vi "LEBITplc.PressureSafety.vi"(0 "i ref in":refnum<vi>, 1 "Nickname in":string, 2 "i attribute in":T1, 3 "value":dbl, 4 "index in":i32, 5 "error in":errorcluster) -> (14 "i ref out":refnum<vi>, 15 "Nickname out":string, 16 "i attribute out":T1, 17 "value out":dbl, 18 "index out":i32, 19 "error out":errorcluster)   [LabVIEW 2014, in "LEBITplc.lvlib"]
uses:
  LEBITplc.lvlib
  LEBITplc.i attribute.ctl
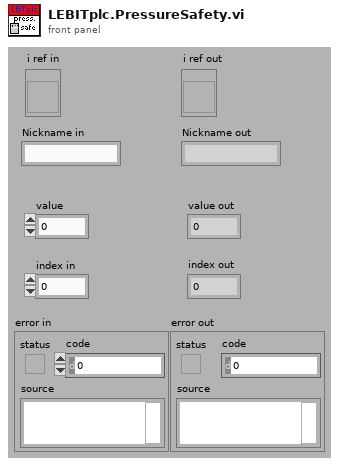
[diagram p1: front panel]
types:
  T1 = typedef "LEBITplc.lvlib/LEBITplc.i attribute.ctl" = cluster{"LLFLocation":string, "SetFileLocation":string, "nickNames":string[], "setValuePLCServiceID":i32[], "GUIServiceID":i32[], "monValuePLC":string[], "SetValueServiceID":i32[], "MonValueServiceID":i32[], "SetValue":dbl[][], "SetValueMin":dbl[], "SetValueMax":dbl[], "SetValueInfoServiceID":i32[], "GUINames":string[], "ListOfBases":string[], "Scale":dbl[], "Offset":dbl[], "setValuePLC":string[], "BaseName":string[], "ScaleServiceID":i32[], "OffsetServiceID":i32[], "AllPLCValues":string[], "CondSpecialArray":string[][], "CondSpecialIndex":i32[], "CondSpecialMonValue":dbl[], "RecentlyChanged":i32[], "SetFileLocationID":i32, "Dependent-Monitors":string[][], "LastLoadedFiles":string[], "IonGuideCalibLocation":string, "Monitor Dependent":string[], "Special":string[], "PLC?":bool[], "Start Date":string, "ListOfBasesServiceID":i32, "SETRA VISA resource":refnum<visa-resource-name>}
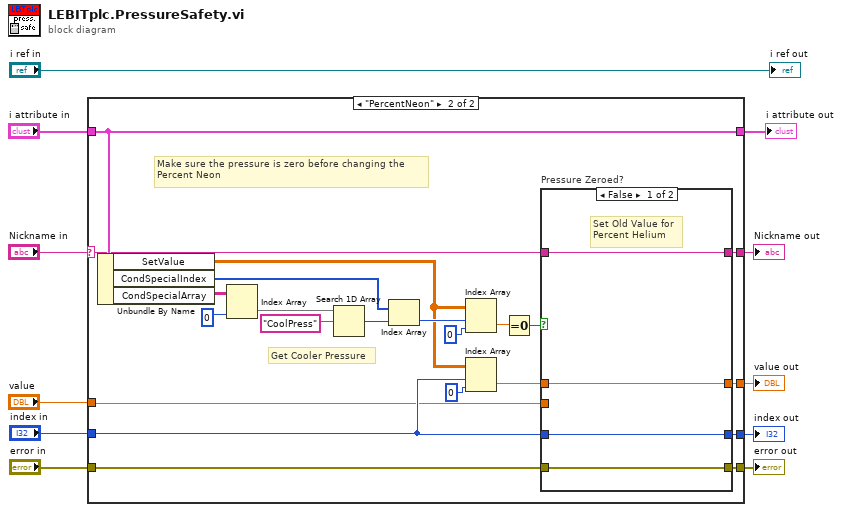
[diagram p0: block diagram]
diagram:
  n1 = case shown="\"PercentNeon\"" "Nickname in" {
    selector: "Nickname in" -> [w14 w34]
    tunnel: "i attribute in" -> [w16 w38]
    tunnel: [w16 w38] -> w9
    tunnel: "value" -> [w13 w20]
    tunnel: [w13 w35] -> w3
    tunnel: [w14 w33] -> w4
    tunnel: "index in" -> [w12 w24]
    tunnel: [w12 w27] -> w2
    tunnel: [w15 w18] -> w5
    tunnel: "error in" -> [w15 w17]
    frame Default {
    }
    frame "PercentNeon" {
      # "Get Cooler Pressure"
      # "Make sure the pressure is zero before changing the \nPercent Neon"
      n2 = Unbundle By Name(w38) -> ("SetValue"=w23:dbl[][], "CondSpecialIndex"=w28:i32[], "CondSpecialArray"=w31:string[][])
      n3 = Index Array(array=w31, index (col)=0 ("index (row)")) -> (element=w32:string[])  [unwired: 1 in]
      n4 = Search 1D Array(1D array=w32, element="CoolPress") -> (index of element=w30:i32)  [unwired: 1 in]
      n5 = Index Array(array=w28, index=w30) -> (element=w29:i32)
      n6 = Index Array(array=w23, index (row)=w29, index (col)=0 ("disabled index (col)")) -> (element=w22:dbl)
      n7 = Index Array(array=w23, index (row)=w24, index (col)=0 ("disabled index (col)")) -> (element=w19:dbl)
      n8 = Equal To 0?(x=w22) -> (x = 0?=w21:bool)
      n9 = case "Pressure Zeroed?" shown="False" w21 {
        tunnel: w20 -> [_ w44]
        tunnel: [w41 w44] -> w35
        tunnel: w34 -> [w40 w45]
        tunnel: [w40 w45] -> w33
        tunnel: [w42 w43] -> w27
        tunnel: w24 -> [w42 w43]
        tunnel: w19 -> [w41 _]
        tunnel: [w39 w46] -> w18
        tunnel: w17 -> [w39 w46]
        frame False {
          # "Set Old Value for\nPercent Helium"
        }
        frame True {
          # "Set New Value for\nPercent Helium"
        }
      }
    }
  }
  "i attribute out" <- w9
  "error out" <- w5
  "Nickname out" <- w4
  "value out" <- w3
  "index out" <- w2
  "i ref out" <- "i ref in"
